vi "NumberDateTimeToSQLDateTime.vi"(9 "StartTime":i32, 11 "StartDate":i32) -> (2 "date/time string":string)   [LabVIEW 2012]
uses:
  <vilib>/Utility/miscctls.llb/LVDateTimeRec.ctl
panel:
  in  "date time rec":T1
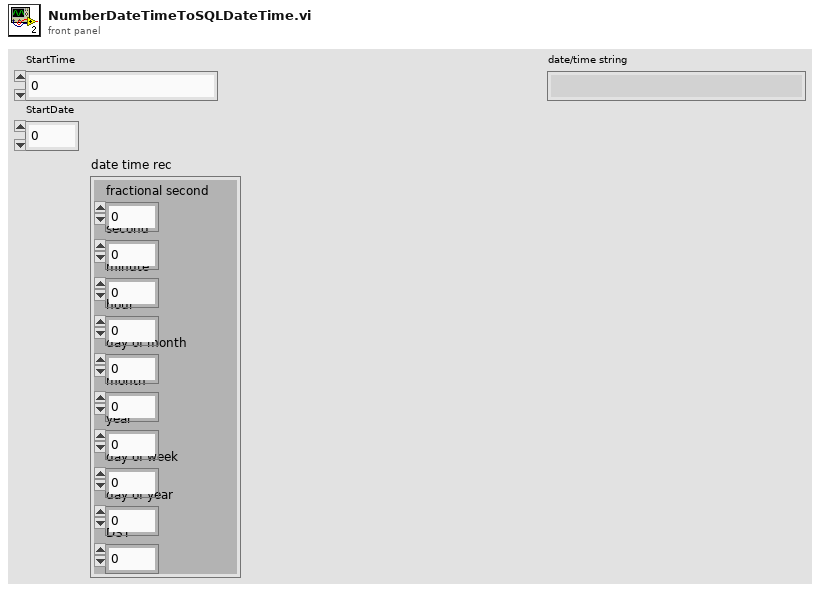
[diagram p1: front panel]
types:
  T1 = typedef "LVDateTimeRec.ctl" = cluster{"fractional second":dbl, "second":i32, "minute":i32, "hour":i32, "day of month":i32, "month":i32, "year":i32, "day of week":i32, "day of year":i32, "DST":i32}
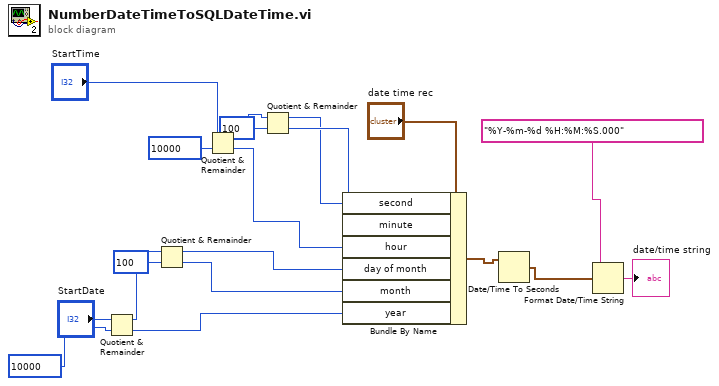
[diagram p0: block diagram]
diagram:
  n1 = Quotient & Remainder(x="StartDate", y=10000) -> (x-y*floor(x/y)=w15:i32, floor(x/y)=w16:i32)
  n2 = Quotient & Remainder(x=w15, y=100) -> (x-y*floor(x/y)=w12:i32, floor(x/y)=w13:i32)
  n3 = Quotient & Remainder(x="StartTime", y=10000) -> (x-y*floor(x/y)=w9:i32, floor(x/y)=w10:i32)
  n4 = Quotient & Remainder(x=w9, y=100) -> (x-y*floor(x/y)=w6:i32, floor(x/y)=w7:i32)
  n5 = Bundle By Name(cluster="date time rec", "second"=w6, "minute"=w7, "hour"=w10, "day of month"=w12, "month"=w13, "year"=w16) -> (w18:T1)
  n6 = Date/Time To Seconds(2:w18) -> (0:w5:timestamp)  [unwired: 1 in]
  n7 = Format Date/Time String(time format string (%c)="%Y-%m-%d %H:%M:%S.000", seconds (now)=w5) -> (date/time string=→"date/time string":string)  [unwired: 1 in]
